vi "Keithley_6514_LabView.vi"() -> ()   [LabVIEW 2024]
panel:
  in  "Volt/Curr":bool
  in  "ProcessFloat":bool=TRUE
  out "Read Data":u32
  out "READ?":u32
  out "READ? and Read Data":u32
  out "number":dbl
  out "substring before match":string
  out "rest of the binary string":string
  in  "byte order (0:big-endian, network order)":T1(ring)=enum."native, host order"
  in  "Boolean":bool=TRUE
  out "value":cluster{dbl}
  out "substring":string
  out "XY Graph":cluster{"Y":dbl[], "Y":dbl[]}[](graph)
  out "timer":u32
  in  "stop":bool
  out "write buffer":string="DISP:DIG 4.5"
  out "error out":errorcluster
  in  "VISA resource name":refnum<visa-resource-name>="GPIB0::14::INSTR"
  in  "access mode":u32
  in  "error in (no error)":errorcluster
  in  "VISA Open timeout (0)":u32
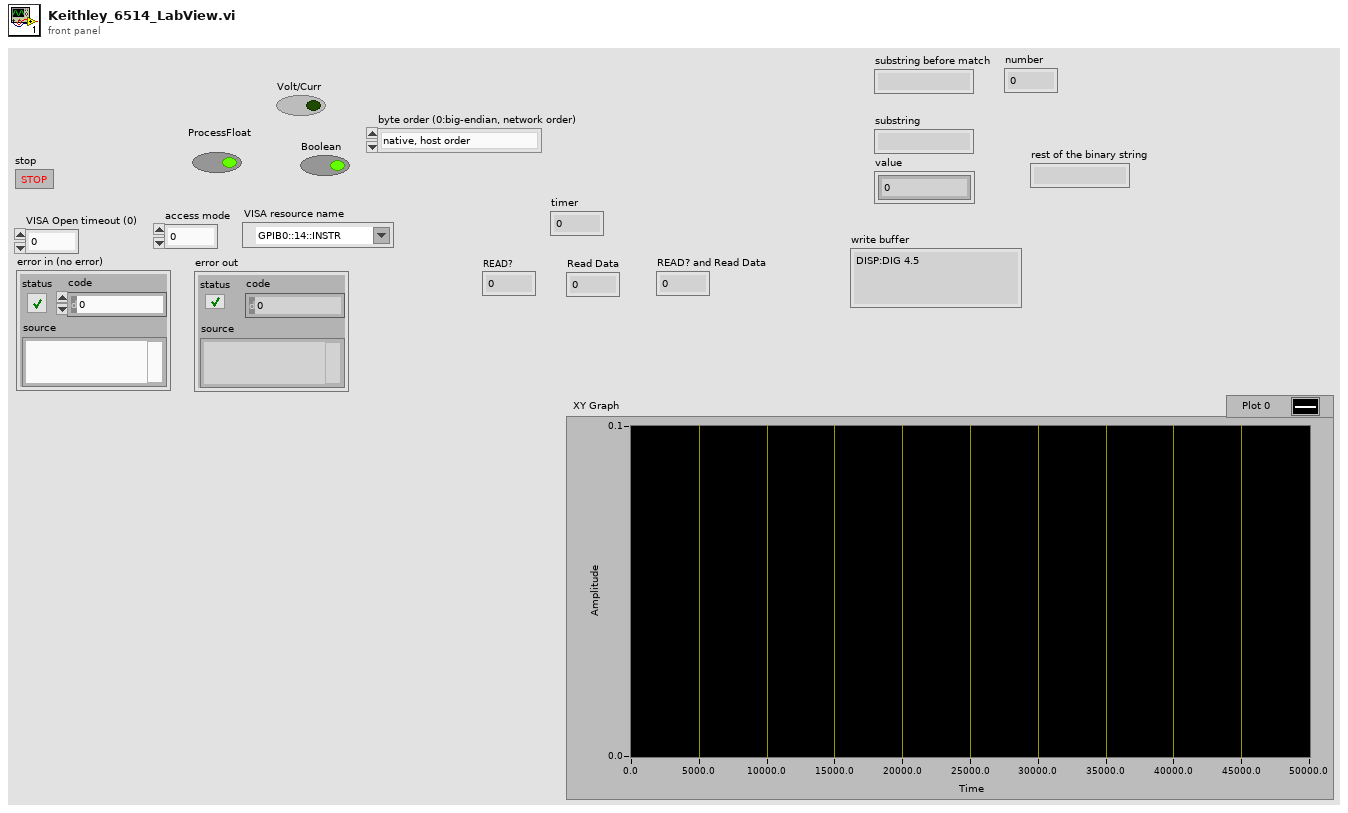
[diagram p1: front panel]
types:
  T1 = enum16{"big-endian, network order", "native, host order", "little-endian"}
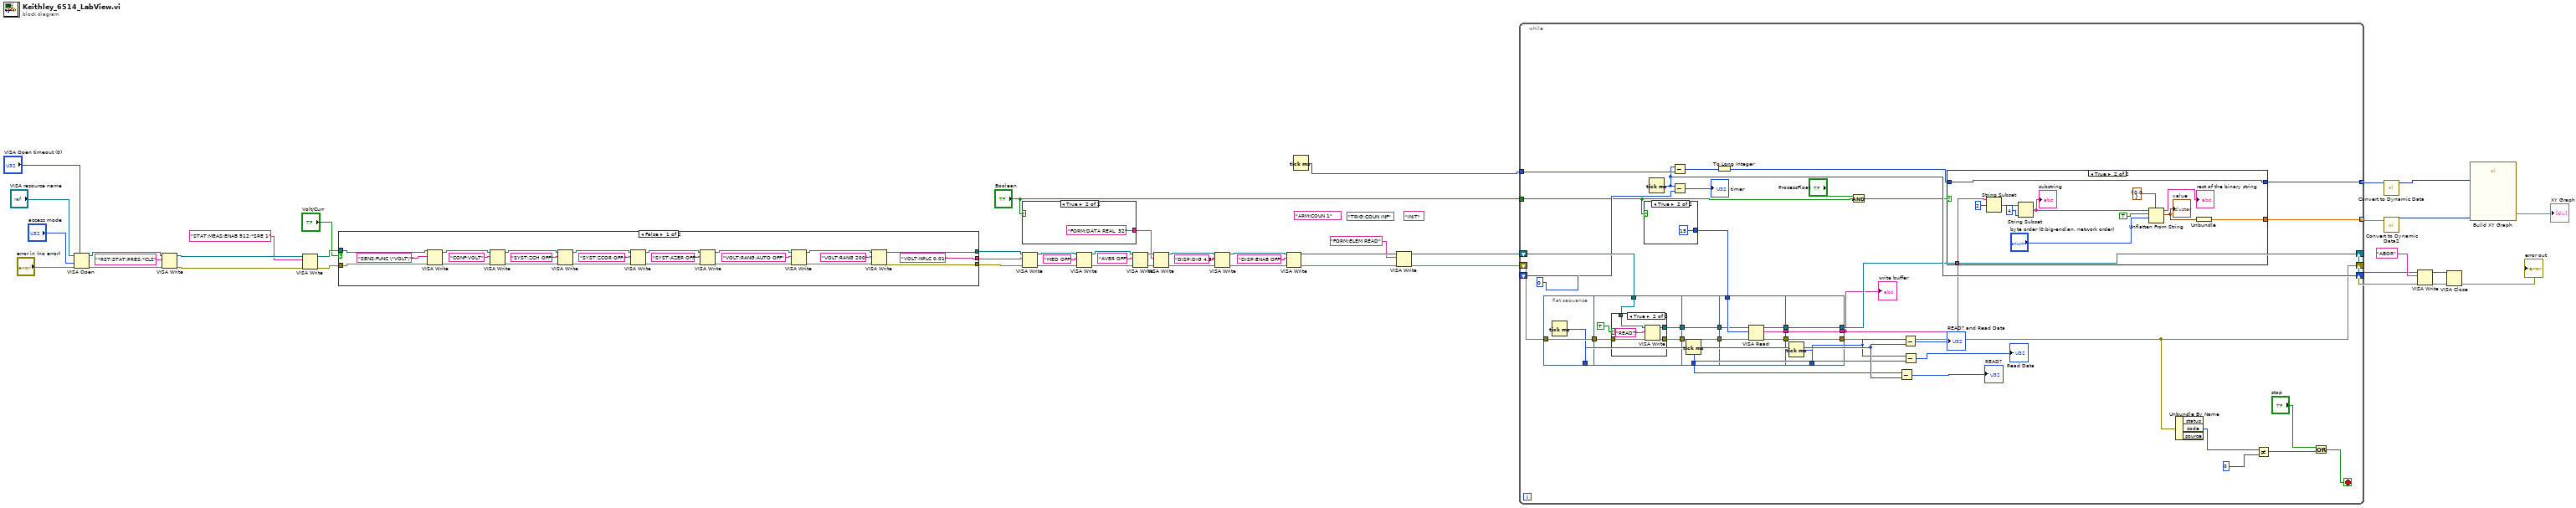
[diagram p0: block diagram]
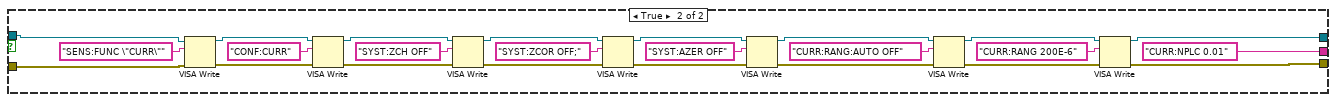
[diagram p2: hidden frame]
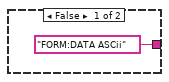
[diagram p3: hidden frame]
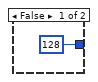
[diagram p5: hidden frame]
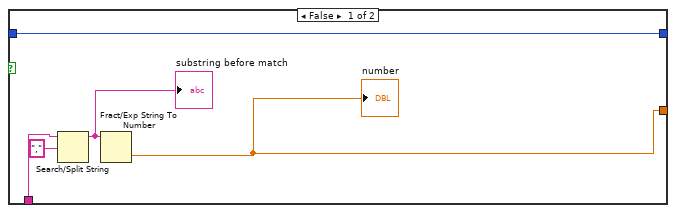
[diagram p6: hidden frame]
diagram:
  (unwired) "INIT" ("write buffer")
  (unwired) "TRIG:COUN INF" ("write buffer")
  (unwired) "ARM:COUN 1" ("write buffer")
  n1 = VISA Open(timeout (0)="VISA Open timeout (0)", access mode="access mode", error in (no error)="error in (no error)", VISA resource name="VISA resource name") -> (VISA resource name=w44:refnum<visa-resource-name>, error out=w45:errorcluster)  [unwired: 1 in]
  n2 = VISA Write(VISA resource name=w44, write buffer="*RST;STAT:PRES;*CLS", error in (no error)=w45) -> (VISA resource name out=w10:refnum<visa-resource-name>, error out=w11:errorcluster)  [unwired: 1 out]
  n3 = VISA Write(VISA resource name=w10, write buffer="STAT:MEAS:ENAB 512;*SRE 1", error in (no error)=w11) -> (VISA resource name out=w8:refnum<visa-resource-name>, error out=w9:errorcluster)  [unwired: 1 out]
  n4 = case shown="False" "Volt/Curr" {
    tunnel: [w53 w79] -> w42
    tunnel: [w51 w78] -> w41
    tunnel: ["VOLT:NPLC 0.01" ("write buffer") "CURR:NPLC 0.01" ("write buffer")] -> w40
    tunnel: w9 -> [w54 w76]
    tunnel: w8 -> [w55 w75]
    frame False {
      n5 = VISA Write(VISA resource name=w55, write buffer="SENS:FUNC \"VOLT\"", error in (no error)=w54) -> (VISA resource name out=w73:refnum<visa-resource-name>, error out=w70:errorcluster)  [unwired: 1 out]
      n6 = VISA Write(VISA resource name=w73, write buffer="CONF:VOLT", error in (no error)=w70) -> (VISA resource name out=w72:refnum<visa-resource-name>, error out=w71:errorcluster)  [unwired: 1 out]
      n7 = VISA Write(VISA resource name=w72, write buffer="SYST:ZCH OFF", error in (no error)=w71) -> (VISA resource name out=w67:refnum<visa-resource-name>, error out=w66:errorcluster)  [unwired: 1 out]
      n8 = VISA Write(VISA resource name=w67, write buffer="SYST:ZCOR OFF;", error in (no error)=w66) -> (VISA resource name out=w57:refnum<visa-resource-name>, error out=w56:errorcluster)  [unwired: 1 out]
      n9 = VISA Write(VISA resource name=w57, write buffer="SYST:AZER OFF", error in (no error)=w56) -> (VISA resource name out=w64:refnum<visa-resource-name>, error out=w61:errorcluster)  [unwired: 1 out]
      n10 = VISA Write(VISA resource name=w64, write buffer="VOLT:RANG:AUTO OFF", error in (no error)=w61) -> (VISA resource name out=w63:refnum<visa-resource-name>, error out=w62:errorcluster)  [unwired: 1 out]
      n11 = VISA Write(VISA resource name=w63, write buffer="VOLT:RANG 200", error in (no error)=w62) -> (VISA resource name out=w53:refnum<visa-resource-name>, error out=w51:errorcluster)  [unwired: 1 out]
    }
    frame True {
      n12 = VISA Write(VISA resource name=w75, write buffer="SENS:FUNC \"CURR\"", error in (no error)=w76) -> (VISA resource name out=w97:refnum<visa-resource-name>, error out=w94:errorcluster)  [unwired: 1 out]
      n13 = VISA Write(VISA resource name=w97, write buffer="CONF:CURR", error in (no error)=w94) -> (VISA resource name out=w96:refnum<visa-resource-name>, error out=w95:errorcluster)  [unwired: 1 out]
      n14 = VISA Write(VISA resource name=w96, write buffer="SYST:ZCH OFF", error in (no error)=w95) -> (VISA resource name out=w91:refnum<visa-resource-name>, error out=w90:errorcluster)  [unwired: 1 out]
      n15 = VISA Write(VISA resource name=w91, write buffer="SYST:ZCOR OFF;", error in (no error)=w90) -> (VISA resource name out=w81:refnum<visa-resource-name>, error out=w80:errorcluster)  [unwired: 1 out]
      n16 = VISA Write(VISA resource name=w81, write buffer="SYST:AZER OFF", error in (no error)=w80) -> (VISA resource name out=w88:refnum<visa-resource-name>, error out=w85:errorcluster)  [unwired: 1 out]
      n17 = VISA Write(VISA resource name=w88, write buffer="CURR:RANG:AUTO OFF", error in (no error)=w85) -> (VISA resource name out=w87:refnum<visa-resource-name>, error out=w86:errorcluster)  [unwired: 1 out]
      n18 = VISA Write(VISA resource name=w87, write buffer="CURR:RANG 200E-6", error in (no error)=w86) -> (VISA resource name out=w79:refnum<visa-resource-name>, error out=w78:errorcluster)  [unwired: 1 out]
    }
  }
  n19 = case shown="True" "Boolean" {
    tunnel: ["FORM:DATA ASCii" ("write buffer") "FORM:DATA REAL, 32" ("write buffer")] -> w17
    frame False {
    }
    frame True {
    }
  }
  n20 = VISA Write(VISA resource name=w42, write buffer=w40, error in (no error)=w41) -> (VISA resource name out=w38:refnum<visa-resource-name>, error out=w37:errorcluster)  [unwired: 1 out]
  n21 = VISA Write(VISA resource name=w38, write buffer="MED OFF", error in (no error)=w37) -> (VISA resource name out=w35:refnum<visa-resource-name>, error out=w34:errorcluster)  [unwired: 1 out]
  n22 = VISA Write(VISA resource name=w35, write buffer="AVER OFF", error in (no error)=w34) -> (VISA resource name out=w27:refnum<visa-resource-name>, error out=w26:errorcluster)  [unwired: 1 out]
  n23 = VISA Write(VISA resource name=w27, write buffer=w17, error in (no error)=w26) -> (VISA resource name out=w29:refnum<visa-resource-name>, error out=w28:errorcluster)  [unwired: 1 out]
  n24 = VISA Write(VISA resource name=w29, write buffer="DISP:DIG 4.5", error in (no error)=w28) -> (VISA resource name out=w32:refnum<visa-resource-name>, error out=w31:errorcluster)  [unwired: 1 out]
  n25 = VISA Write(VISA resource name=w32, write buffer="DISP:ENAB OFF", error in (no error)=w31) -> (VISA resource name out=w5:refnum<visa-resource-name>, error out=w2:errorcluster)  [unwired: 1 out]
  n26 = Tick Count (ms)() -> (millisecond timer value=w24:u32)
  n27 = VISA Write(VISA resource name=w5, write buffer="FORM:ELEM READ", error in (no error)=w2) -> (VISA resource name out=w4:refnum<visa-resource-name>, error out=w3:errorcluster)  [unwired: 1 out]
  n28 = while {
    shift-right: [w129] -> w13
    shift-left: w4 -> [w136]
    shift-right: [w104] -> w12
    shift-left: w3 -> [w135]
    shift-right: [w131] -> _
    shift-left: u32 0 ("millisecond timer value") -> [w134]
    tunnel: w24 -> [w132]
    tunnel: [w127] -> w22 mode=indexing
    tunnel: [w126] -> w21 mode=indexing
    tunnel: "Boolean" -> [w109]
    stop <- w101 stop-if-true
    n29 = flat-sequence {
      tunnel: w135 -> [w138]
      tunnel: [w138] -> w125
      tunnel: [w137] -> w119
      tunnel: w136 -> [w143]
      tunnel: w125 -> [w142]
      tunnel: [w141] -> w117
      tunnel: [w140] -> w115
      tunnel: w117 -> [w153]
      tunnel: [w153] -> w116
      tunnel: w115 -> [w152]
      tunnel: [w152] -> w114
      tunnel: [w151] -> w112
      tunnel: [w156] -> w123
      tunnel: [w154] -> w122
      tunnel: [w155] -> w121
      tunnel: w116 -> [w159]
      tunnel: w120 -> [w158]
      tunnel: w114 -> [w157]
      tunnel: [w161] -> w107
      tunnel: [w162] -> w129
      tunnel: [w163] -> w104
      tunnel: w123 -> [w163]
      tunnel: w122 -> [w162]
      tunnel: w121 -> [w161]
      tunnel: [w160] -> w113
      frame #0 {
        n30 = Tick Count (ms)() -> (millisecond timer value=w137:u32)
      }
      frame #1 {
        n31 = case shown="True" TRUE {
          tunnel: w143 -> [w144 w150]
          tunnel: w142 -> [w145 w149]
          tunnel: [w145 w147] -> w141
          tunnel: [w144 w146] -> w140
          frame False {
          }
          frame True {
            n32 = VISA Write(VISA resource name=w150, write buffer="READ?", error in (no error)=w149) -> (VISA resource name out=w146:refnum<visa-resource-name>, error out=w147:errorcluster)  [unwired: 1 out]
          }
        }
      }
      frame #2 {
        n33 = Tick Count (ms)() -> (millisecond timer value=w151:u32)
      }
      frame #3 {
        n34 = VISA Read(VISA resource name=w157, byte count=w158, error in (no error)=w159) -> (VISA resource name out=w154:refnum<visa-resource-name>, read buffer=w155:string, error out=w156:errorcluster)  [unwired: 1 out]
      }
      frame #4 {
        n35 = Tick Count (ms)() -> (millisecond timer value=w160:u32)
      }
    }
    n36 = case shown="True" w109 {
      tunnel: [u32 128 ("byte count") u32 15 ("byte count")] -> w120
      frame False {
      }
      frame True {
      }
    }
    n37 = Tick Count (ms)() -> (millisecond timer value=w131:u32)
    n38 = Subtract(x=w131, y=w132) -> (x-y=w130:u32)
    n39 = Subtract(x=w131, y=w134) -> (x-y=→"timer":u32)
    n40 = To Long Integer(number=w130) -> (32bit integer=w128:i32)
    n41 = And(x="ProcessFloat", y=w109) -> (x .and. y?=w110:bool)
    n42 = Subtract(x=w112, y=w119) -> (x-y=→"READ?":u32)
    n43 = Subtract(x=w113, y=w119) -> (x-y=→"READ? and Read Data":u32)
    n44 = Subtract(x=w113, y=w112) -> (x-y=→"Read Data":u32)
    n45 = case shown="True" w110 {
      tunnel: w128 -> [w170 w174]
      tunnel: [w166 w172] -> w127
      tunnel: [w170 w174] -> w126
      tunnel: w107 -> [w168 w171]
      frame False {
        n46 = Search/Split String(string=w168, search string/char (-)=",") -> (substring before match=w167:string)  [unwired: 1 in, 2 out]
        "substring before match" <- w167
        n47 = Fract/Exp String To Number(string=w167) -> (number=w166:dbl)  [unwired: 3 in, 1 out]
        "number" <- w166
      }
      frame True {
        n48 = String Subset(string=w171, offset (0)=2 ("length (rest)")) -> (substring=w176:string)  [unwired: 1 in]
        n49 = String Subset(string=w176, length (rest)=4 ("length (rest)")) -> (substring=w177:string)  [unwired: 1 in]
        "substring" <- w177
        n50 = Unflatten From String(type=cluster{sgl} {0.0}, binary string=w177, data includes array or string size? (T)=TRUE, byte order (0:big-endian, network order)="byte order (0:big-endian, network order)") -> (rest of the binary string=→"rest of the binary string":string, value=w173:cluster{sgl})  [unwired: 1 in, 1 out]
        "value" <- w173
        n51 = Unbundle(w173) -> (w172:sgl)
      }
    }
    n52 = Unbundle By Name(w104) -> ("code"=w103:i32)  [unwired: 2 out]
    n53 = Not Equal?(x=w103, y=0) -> (x != y?=w105:bool)
    n54 = Or(x="stop", y=w105) -> (x .or. y?=w101:bool)
    "write buffer" <- w107
  }
  n55 = call "Convert to Dynamic Data"("Array"=w21) -> ("Dynamic Data Type"=w20:dynamicdata)  [unwired: 3 in]
  n56 = call "Convert to Dynamic Data2"("Array"=w22) -> ("Dynamic Data Type"=w19:dynamicdata)  [unwired: 3 in]
  n57 = VISA Write(VISA resource name=w13, write buffer="ABOR", error in (no error)=w12) -> (VISA resource name out=w15:refnum<visa-resource-name>, error out=w14:errorcluster)  [unwired: 1 out]
  n58 = VISA Close(VISA resource name=w15, error in (no error)=w14) -> (error out=→"error out":errorcluster)
  n59 = call "Build XY Graph"("Y Input"=w19, "X Input"=w20) -> ("XY Graph"=→"XY Graph":cluster{"X":dbl[], "Y":dbl[]}[])  [unwired: 8 in, 1 out]
